vi "IMAQDevice.ProcPeriodic.vi"(0 "i ref in":refnum<vi>, 3 "ms timeout (10000)":i32=10000, 5 "error in (no error)":errorcluster) -> (14 "i ref out":refnum<vi>, 17 "timed out":bool, 19 "error out":errorcluster)   [LabVIEW 2014, in "IMAQDevice.lvlib"]
doc: "This method serves to periodically do things like reading values from the HW. Methods that should be executed periodically should be called from THIS methode. Add code here."
uses:
  IMAQDevice.lvlib
  CSlibraries-extern/DimLVEvent/LVDimInterface/LVDimInterface.lvlib
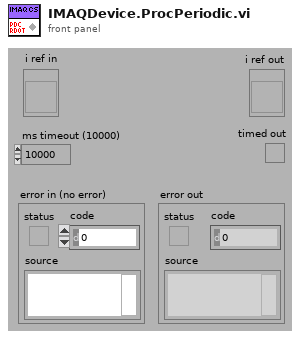
[diagram p1: front panel]
types:
  T1 = typedef "IMAQDevice.lvlib/IMAQDevice.i attribute.ctl" = cluster{"HGF_IMAQ.lvlib:HGF_IMAQDevice.lvclass":refnum<class "HGF_IMAQDevice.lvclass">, "Image":T2, "TimeStampID":i32, "Image IDs":i32[], "NumberOfImagesID":i32, "JPEG?":bool, "JPEGID":i32, "JPEG_ImageID":i32, "TriggerModeID":i32, "OffsetFromLeft":i32, "OffsetFromTop":i32, "HorizontalPixelPerMm":dbl, "VerticalPixelPerMm":dbl, "Grid":cluster{"1":cluster{i32, i32}, "2":cluster{i32, i32}, "3":cluster{i32, i32}, "4":cluster{i32, i32}}, "GridR":cluster{"1":cluster{dbl, dbl}, "2":cluster{dbl, dbl}, "3":cluster{dbl, dbl}, "4":cluster{dbl, dbl}}, "CameraTypeID":i32, "CameraInfos":cluster{"Camera Name-Array":string[], "own Camera Type":string}, "TakeMeasurement?":bool, "TriggerArmedID":i32, "Mirroring":i16, "Rotation":dbl}
  T2 = typedef "IMAQ Image.ctl" = refnum<image>
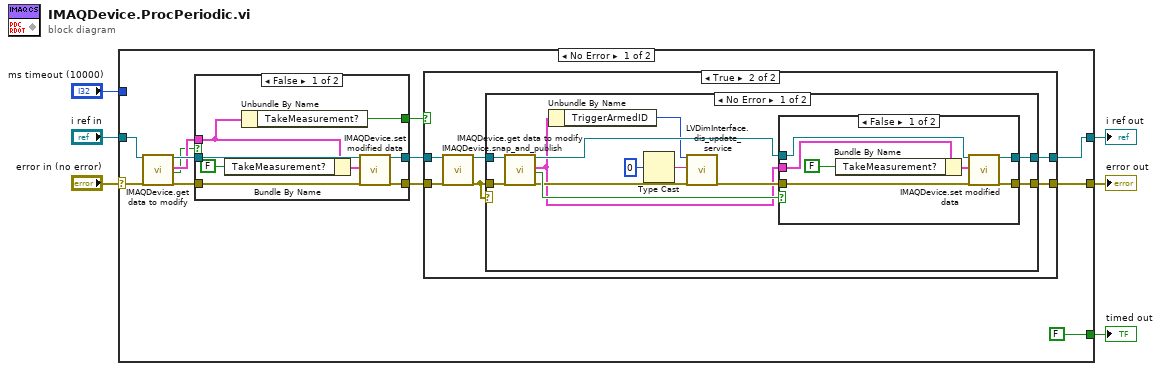
[diagram p0: block diagram]
diagram:
  n1 = case shown="No Error" "error in (no error)" {
    selector: "error in (no error)" -> [w15 w60]
    tunnel: [w16 w60] -> w5
    tunnel: "i ref in" -> [w14 w61]
    tunnel: [w17 w61] -> w3
    tunnel: [FALSE _] -> w2
    tunnel: "ms timeout (10000)" -> [_ _]
    frame No Error {
      n2 = call "IMAQDevice.get data to modify.vi"("i ref in"=w14, "error in (no error)"=w15) -> ("i ref out"=w12:refnum<vi>, "i attribute"=w9:T1, "timed out"=w8:bool, "error out"=w13:errorcluster)  [unwired: 14 in]
      n3 = case shown="False" w8 {
        tunnel: w13 -> [w26 w27]
        tunnel: w12 -> [w25 w28]
        tunnel: [w24 w28] -> w11
        tunnel: [w23 w27] -> w10
        tunnel: w9 -> [w20 _]
        tunnel: [w19 _] -> w7
        frame False {
          n4 = Bundle By Name(cluster=w20, "TakeMeasurement?"=FALSE) -> (w22:T1)
          n5 = Unbundle By Name(w20) -> ("TakeMeasurement?"=w19:bool)
          n6 = call "IMAQDevice.set modified data.vi"("i ref in"=w25, "i attribute"=w22, "error in (no error)"=w26) -> ("i ref out"=w24:refnum<vi>, "error out"=w23:errorcluster)  [unwired: 15 in]
        }
        frame True {
        }
      }
      n7 = case shown="True" w7 {
        tunnel: w11 -> [w29 w36]
        tunnel: [w29 w33] -> w17
        tunnel: w10 -> [w30 w35]
        tunnel: [w30 w31] -> w16
        frame False {
        }
        frame True {
          n8 = call "IMAQDevice.snap_and_publish.vi"("i ref in"=w36, "error in (no error)"=w35) -> ("i ref out"=w34:refnum<vi>, "error out"=w32:errorcluster)  [unwired: 16 in]
          n9 = case shown="No Error" w32 {
            tunnel: w34 -> [w48 w58]
            tunnel: w32 -> [w47 w59]
            tunnel: [w45 w58] -> w33
            tunnel: [w44 w59] -> w31
            frame No Error {
              n10 = call "IMAQDevice.get data to modify.vi"("i ref in"=w48, "error in (no error)"=w47) -> ("i ref out"=w40:refnum<vi>, "i attribute"=w38:T1, "timed out"=w46:bool, "error out"=w42:errorcluster)  [unwired: 14 in]
              n11 = Unbundle By Name(w38) -> ("TriggerArmedID"=w37:i32)
              n12 = Type Cast(x=0) -> (*(type *) &x=w39:string)  [unwired: 1 in]
              n13 = call "LVDimInterface.dis_update_service.vi"("my_serviceID"=w37, "data"=w39, "error in (no error)"=w42) -> ("error out"=w41:errorcluster)  [unwired: 14 in, 2 out]
              n14 = case shown="False" w46 {
                tunnel: w41 -> [w55 w56]
                tunnel: [w54 w56] -> w44
                tunnel: w40 -> [w53 w57]
                tunnel: [w52 w57] -> w45
                tunnel: w38 -> [w50 _]
                frame False {
                  n15 = Bundle By Name(cluster=w50, "TakeMeasurement?"=FALSE) -> (w51:T1)
                  n16 = call "IMAQDevice.set modified data.vi"("i ref in"=w53, "i attribute"=w51, "error in (no error)"=w55) -> ("i ref out"=w52:refnum<vi>, "error out"=w54:errorcluster)  [unwired: 15 in]
                }
                frame True {
                }
              }
            }
            frame Error {
            }
          }
        }
      }
    }
    frame Error {
    }
  }
  "error out" <- w5
  "i ref out" <- w3
  "timed out" <- w2
